vi "ExpressAbilitySub_OnLocaleChange.vi"(7 "State In":T1 {"BlockNodeState"."Draw Style" items=["FunctionBlock", "ExpressVI", "Variable", "Elemental I/O", "32x32 Icon", "FunctionBlockCompact"]; "BlockNodeState"."Terminal Data"."Terminal Flags" format="%.0b"}) -> (8 "State Out":T1 {"BlockNodeState"."Draw Style" items=["FunctionBlock", "ExpressVI", "Variable", "Elemental I/O", "32x32 Icon", "FunctionBlockCompact"]; "BlockNodeState"."Terminal Data"."Terminal Flags" format="%.0b"})   [LabVIEW 2017]
uses:
  <vilib>/express/express shared/XNodes/controls/ExpressBlockNodeState.ctl
  <vilib>/BlockNodeSupport/BlockNodeState.ctl
  <vilib>/BlockNodeSupport/TerminalData.ctl
  <vilib>/picture/picture.llb/imagedata.ctl
  <vilib>/express/express shared/XNodes/controls/ExpressState.ctl
  <vilib>/express/express shared/XNodes/controls/ExpressTerminalInfo.ctl
  <vilib>/XNodeSupport/XNodeType.ctl
  <vilib>/XNodeSupport/NI_XNodeSupport.lvlib
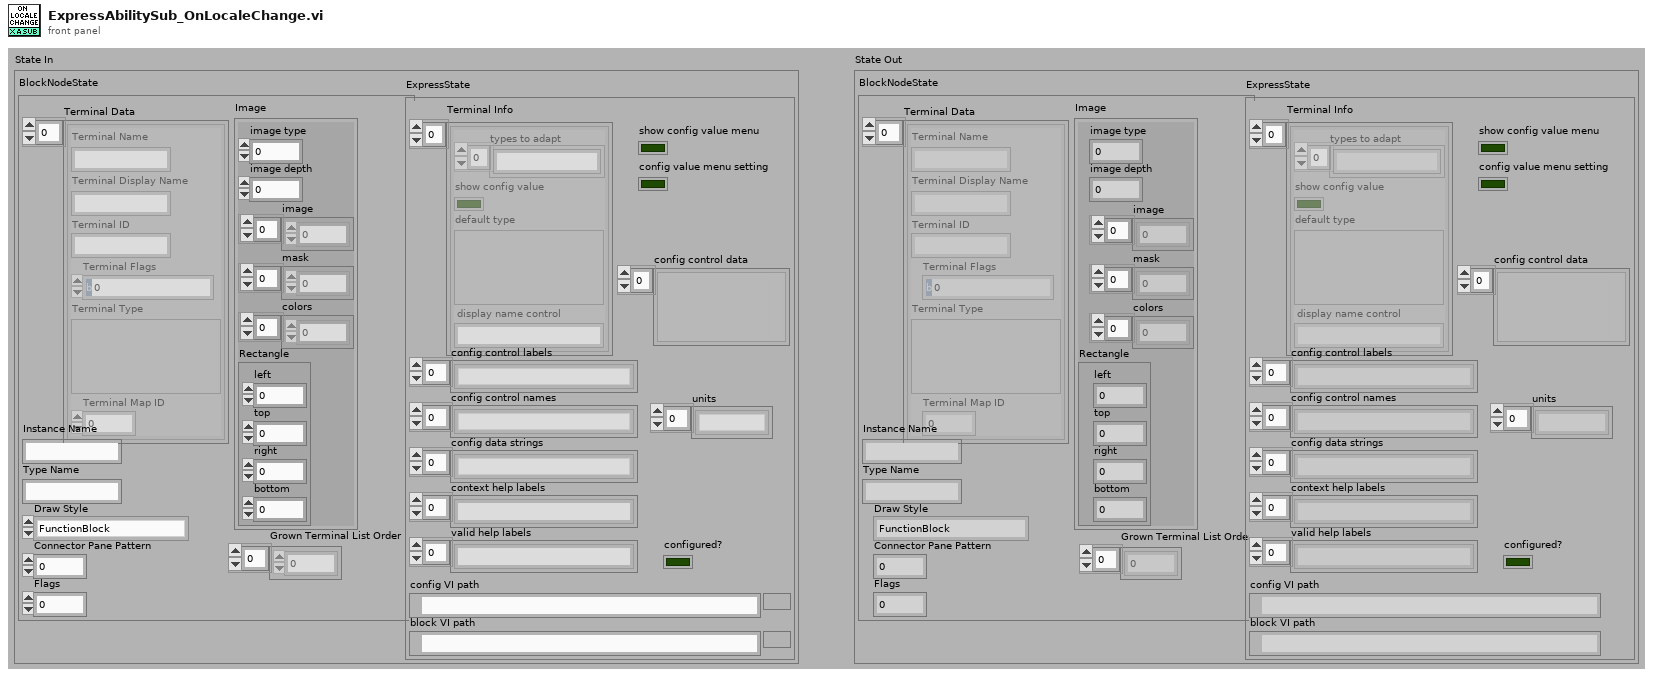
[diagram p1: front panel]
types:
  T1 = typedef "ExpressBlockNodeState.ctl" = cluster{"BlockNodeState":T2, "ExpressState":T5}
  T2 = typedef "BlockNodeState.ctl" = cluster{"Terminal Data":T3[], "Instance Name":string, "Type Name":string, "Draw Style":i32, "Connector Pane Pattern":i32, "Flags":i32, "Grown Terminal List Order":i32[], "Image":T4}
  T3 = typedef "TerminalData.ctl" = cluster{"Terminal Name":string, "Terminal Display Name":string, "Terminal ID":string, "Terminal Flags":i32, "Terminal Type":variant, "Terminal Map ID":i32}
  T4 = typedef "imagedata.ctl" = cluster{"image type":i32, "image depth":i32, "image":u8[], "mask":u8[], "colors":u32[], "Rectangle":cluster{"left":i16, "top":i16, "right":i16, "bottom":i16}}
  T5 = typedef "ExpressState.ctl" = cluster{"Terminal Info":T6, "config control names":string[], "config data strings":string[], "config control data":variant[], "units":string[], "configured?":bool, "config VI path":path, "block VI path":path, "config control labels":string[], "show config value menu":bool, "config value menu setting":bool, "context help labels":string[], "valid help labels":string[]}
  T6 = typedef "ExpressTerminalInfo.ctl" = cluster{"types to adapt":string[], "show config value":bool, "default type":T7, "display name control":string}[]
  T7 = typedef "NI_XNodeSupport.lvlib/XNodeType.ctl" = variant
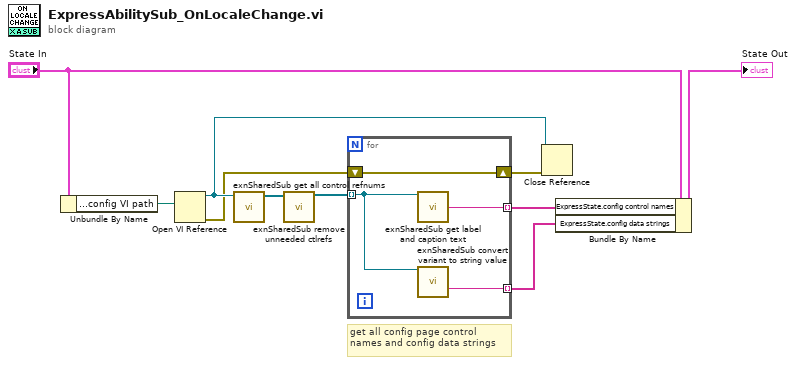
[diagram p0: block diagram]
diagram:
  # "get all config page control names and config data strings"
  n1 = Unbundle By Name("State In") -> ("ExpressState.config VI path"=w1:path)
  n2 = Open VI Reference(vi path=w1) -> (vi reference=w10:refnum<vi>, error out=w4:errorcluster)  [unwired: 5 in]
  n3 = call <vilib>:"exnSharedSub get all control refnums.vi"("viref Express VI"=w10) -> ("All Controls[]"=w2:refnum<vi>[])  [unwired: 2 in, 1 out]
  n4 = call <vilib>:"exnSharedSub remove unneeded ctlrefs.vi"("Ctl Refnums in"=w2) -> ("Ctl Refnums out"=w3:refnum<vi>[])  [unwired: 14 in]
  n5 = for {
    tunnel: w3 -> [w12] mode=indexing
    shift-right: [w14] -> w9
    shift-left: w4 -> [w14]
    tunnel: [w11] -> w5 mode=indexing
    tunnel: [w13] -> w6 mode=indexing
    n6 = call <vilib>:"exnSharedSub get label and caption text.vi"("control reference"=w12) -> ("base name"=w11:string)  [unwired: 12 in, 2 out]
    n7 = call <vilib>:"exnSharedSub convert variant to string value.vi"("control reference"=w12) -> ("string value"=w13:string)  [unwired: 13 in, 1 out]
  }
  n8 = Close Reference(reference=w10, error in (no error)=w9) -> ()  [unwired: 1 out]
  n9 = Bundle By Name(cluster="State In", "ExpressState.config control names"=w5, "ExpressState.config data strings"=w6) -> (→"State Out":T1)
